vi "NLEISView_Subvi_v15.vi"(0 "Ratio Multiplier":dbl=1.5, 1 "Vk Fitting Algorithm":string(combo)="0", 2 "Char Current (Amps)":dbl=0.067 format="%.5f", 3 "file path (dialog if empty)":path, 4 "LS Program":bool, 5 "Sigma Multiplier":dbl=1.5, 7 "Vk Fitting Tolerance":dbl=0.0001, 9 "Amplitude Run Number":i32, 11 "Frequency Run Number":i32, 12 "Gaussian Window\nParameter (B)":dbl=20.0, 14 "Lookup Table":dbl[][](array[numeric]), 15 "Perturbation Method":bool) -> (6 "Frequency":sgl format="%#.6f", 10 "Fit Coefficients and Noise Ratios":dbl[](array[numeric]) format="%.2f")   [LabVIEW 2018]
uses:
  <vilib>/Analysis/baseanly.llb/Mean (DBL).vi
  <vilib>/Analysis/5stat.llb/RMS (DBL).vi
  <vilib>/Utility/file.llb/Read From Spreadsheet File (DBL).vi
  <vilib>/measure/maspectr.llb/FFT Spectrum (Mag-Phase) for 1 Chan.vi
  <vilib>/Waveform/WDTOps.llb/WDT Get Waveform Time Array DBL.vi
  <vilib>/measure/maspectr.llb/FFT Spectrum (Real-Im) for 1 Chan.vi
  <vilib>/measure/NI_MAPro.lvlib
  <vilib>/Analysis/NI_AALPro.lvlib
  <vilib>/Analysis/NI_AALBase.lvlib
panel:
  out "Voltage (Re and Im), Gaussian FFT vs Fit":dbl[][](graph)
  out "Current (Re and Im), Gaussian FFT vs Fit":dbl[][](graph)
  out "Pre-Filter":dbl[](array[numeric])
  in  "Tab Control":enum32{"Fitting", "Data"}(tab)
  out "sigma noise":dbl format="%.5e"
  out "Current Amplitude":dbl format="%.3f"
  out "V1 Amplitude":dbl format="%.2f"
  out "Current Phase Correction":dbl
  out "Voltage vs Time":cluster{dbl[], dbl[]}(graph)
  out "Current vs Time":cluster{dbl[], dbl[]}(graph)
  out "Current vs Time (Gaussian Window)":waveform(dbl)(graph)
  out "Post-Filter":dbl[](array[numeric])
  out "Voltage Magnitude Hanning FFT":cluster{"f0":dbl, "df":dbl, "magnitude":dbl[]}(graph)
  out "Current Magnitude Hanning FFT":cluster{"f0":dbl, "df":dbl, "magnitude":dbl[]}(graph)
  out "Voltage vs Time (Gaussian Window)":waveform(dbl)(graph)
  # "Fit Voltage Coefficients"
  # "V1 Re\nV1 Im"
  # "V2 Re\nV2 Im"
  # "V3 Re\nV3 Im"
  # "V4 Re\nV4 Im"
  # "V5 Re\nV5 Im"
  # "Flat Baseline Im\nFlat Baseline Re"
  # "Sloped Baseline Origin\nSloped Baseline End"
  # "Appended Array Built As:\n0 - alpha\n1 - V1 Re\n2 - V1 Im\n3 - V2 Re\n4 - V2 Im\n5 - V3 Re\n6 - V3 Im\n7 - V4 Re\n8 - V4 Im\n9 - V5 Re\n10 - V5 Im\n11 - V1 Mag\n12 - V2 Mag\n13 - V3 Mag\n14 - V4 Mag\n15 - V5 Mag\n16 - V1 Phase\n17 - V2 Phase\n18 - V3 Phase\n19 - V4 Phase\n20 - V5 Phase\n21 - alpha Peak/Noise (rms/sigma)\n22 - alpha Noise/Error\n23 - V1 Peak/Noise\n24 - V1 Noise/Error\n25 - V2 Peak/Noise\n26 - V2 Noise/Error\n27 - V3 Peak/Noise\n28 - V3 Noise/Error\n29 - V4 Peak/Noise\n30 - V4 Noise/Error\n31 - V5 Peak/Noise\n32 - V5 Noise/Error"
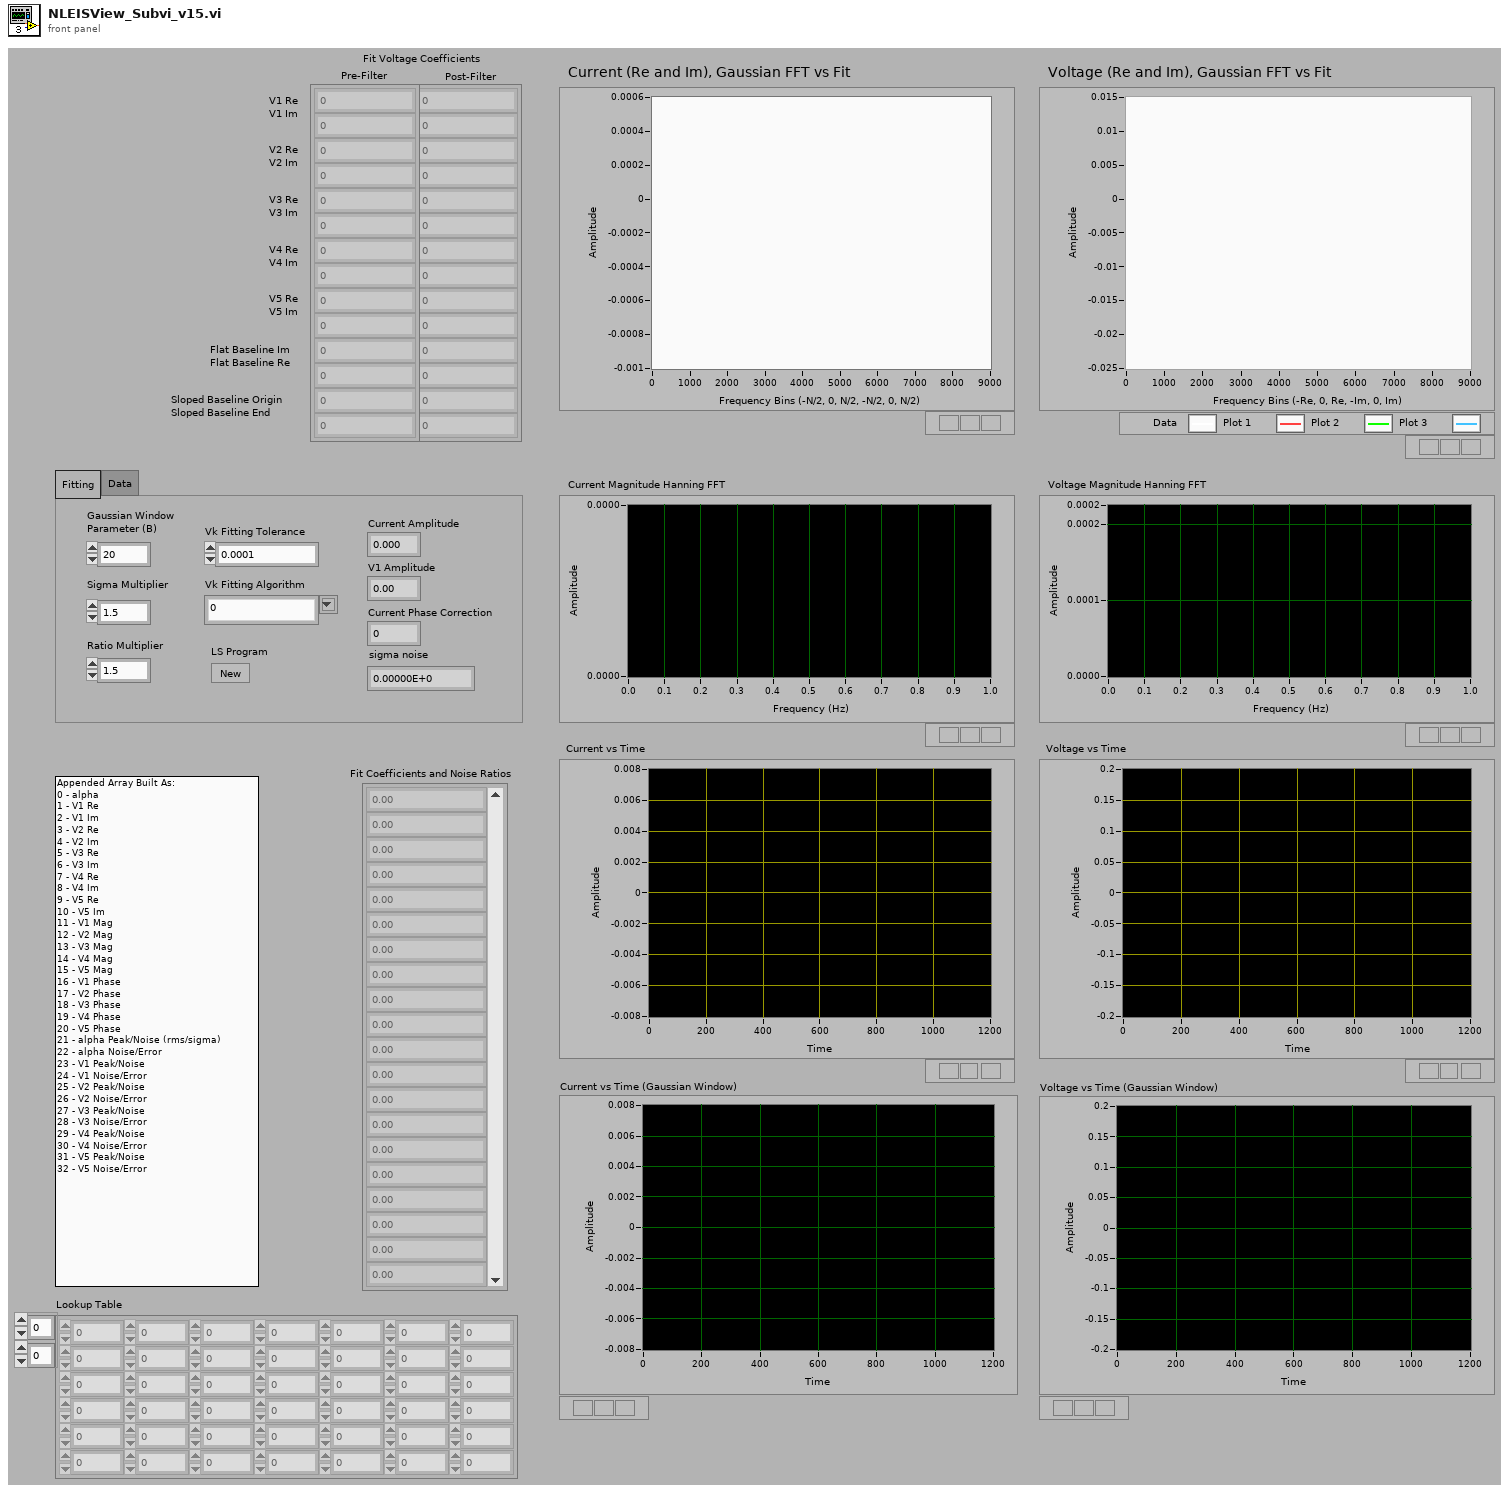
[diagram p1: front panel]
types:
  T1 = enum16{"None ", "Hanning", "Hamming", "Blackman-Harris", "Exact Blackman", "Blackman", "Flat Top", "4 Term B-Harris ", "7 Term B-Harris", "Low Sidelobe"}
  T2 = cluster{"f0":dbl, "df":dbl, "imaginary part":dbl[]}
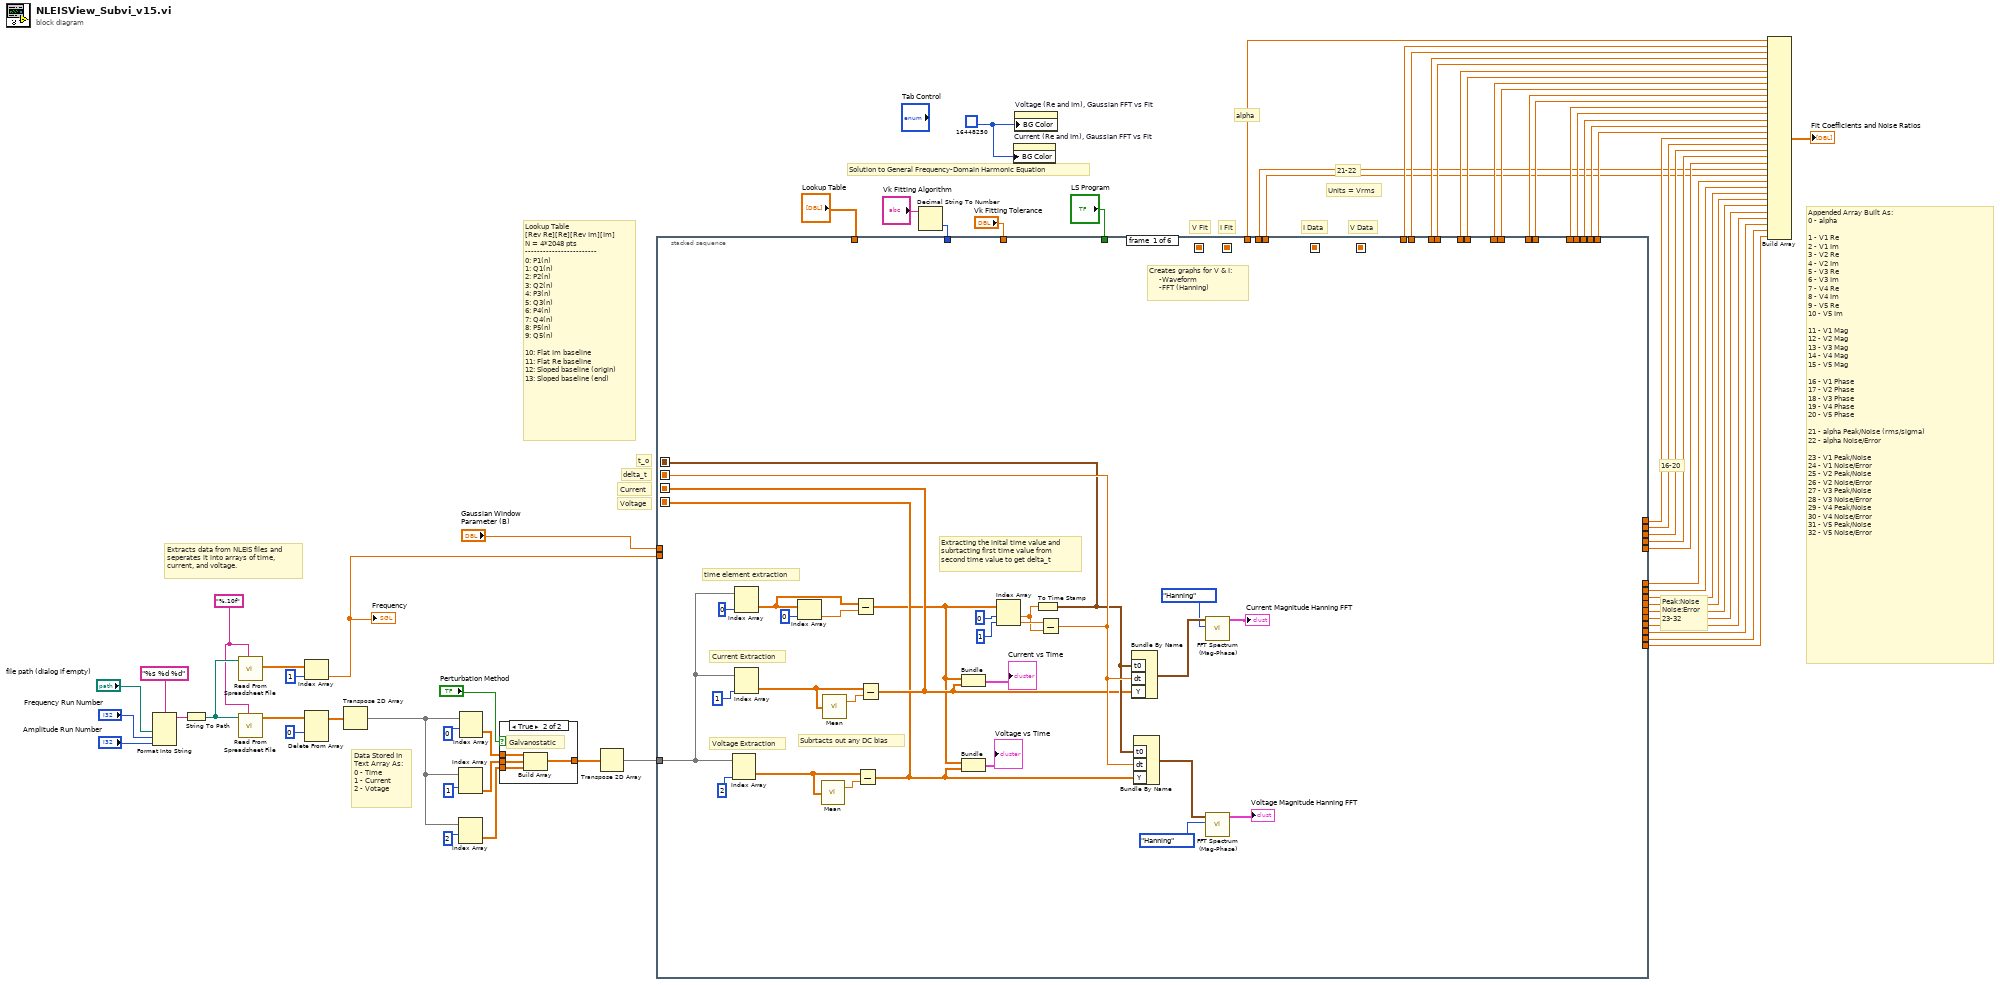
[diagram p0: block diagram]
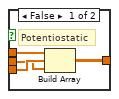
[diagram p2: hidden frame]
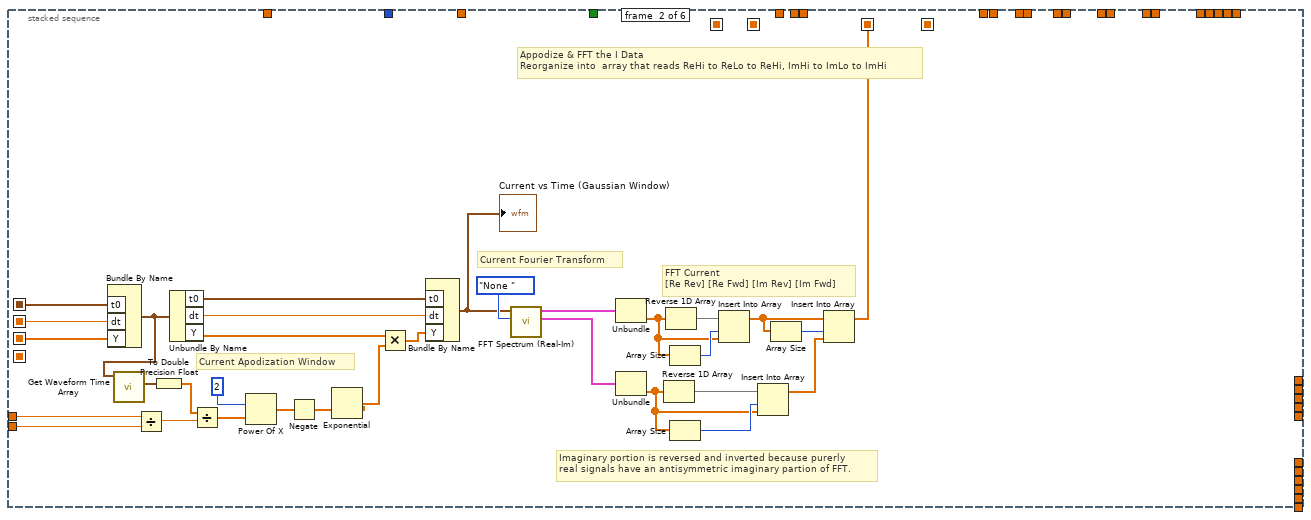
[diagram p3: hidden frame]
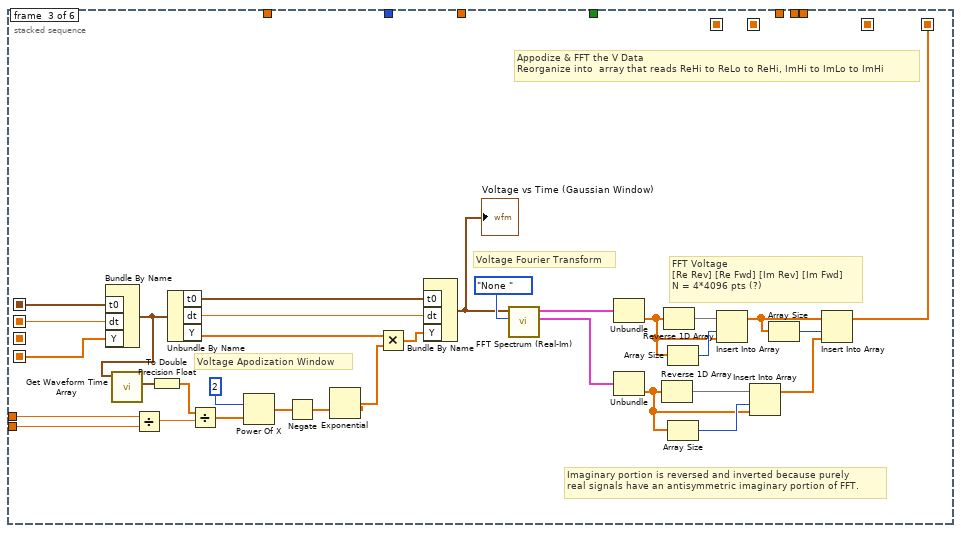
[diagram p4: hidden frame]
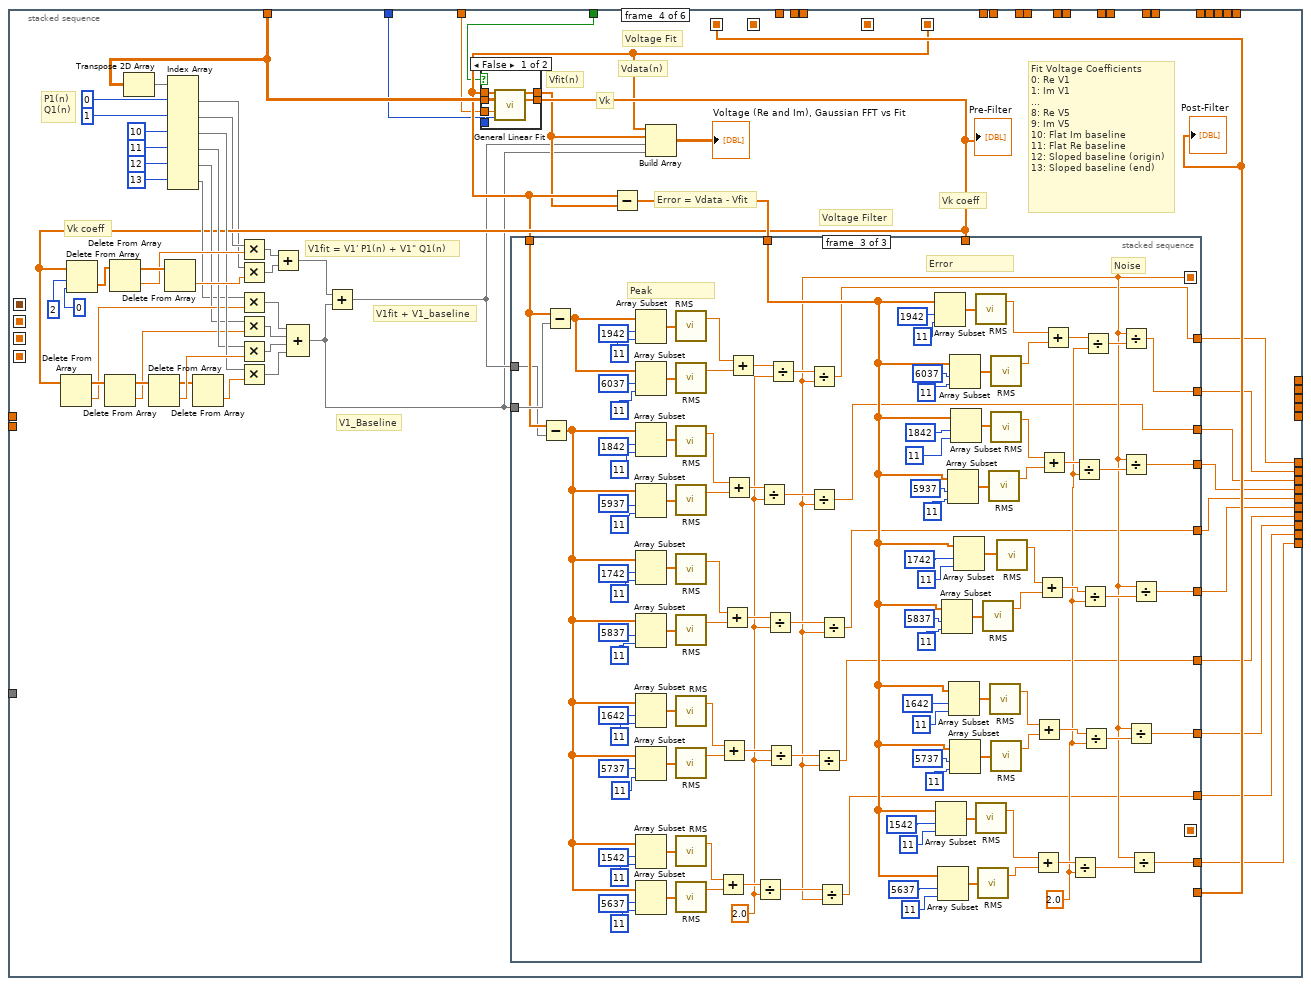
[diagram p5: hidden frame]
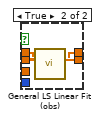
[diagram p6: hidden frame]
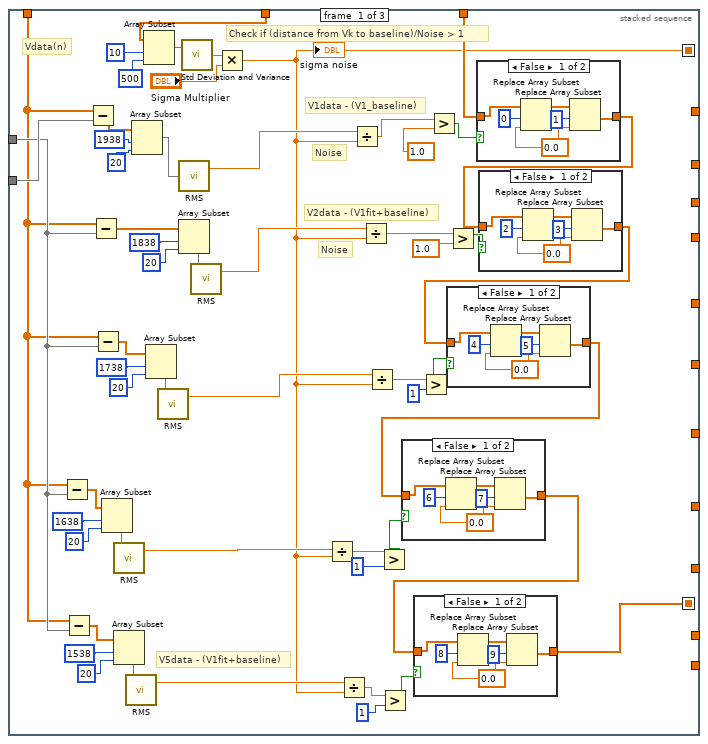
[diagram p7: hidden frame]
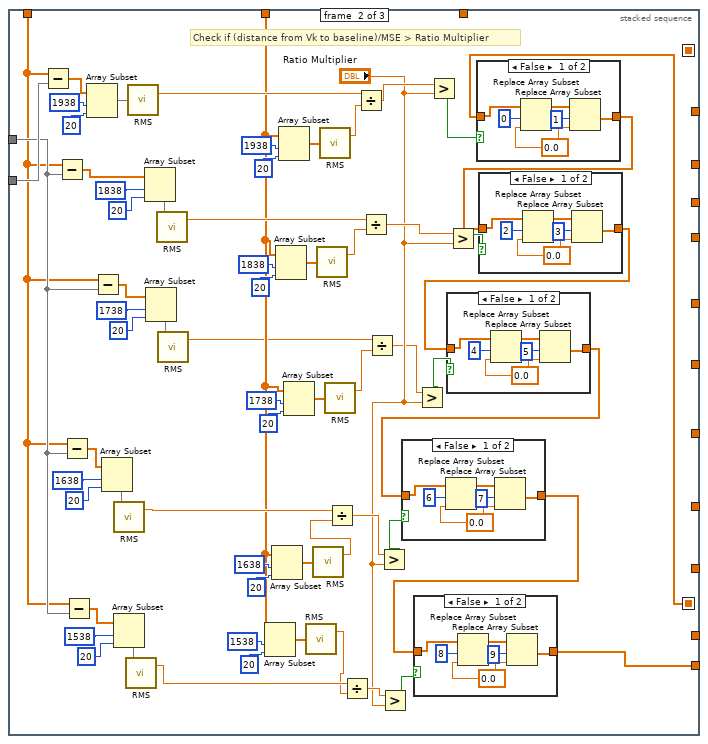
[diagram p13: hidden frame]
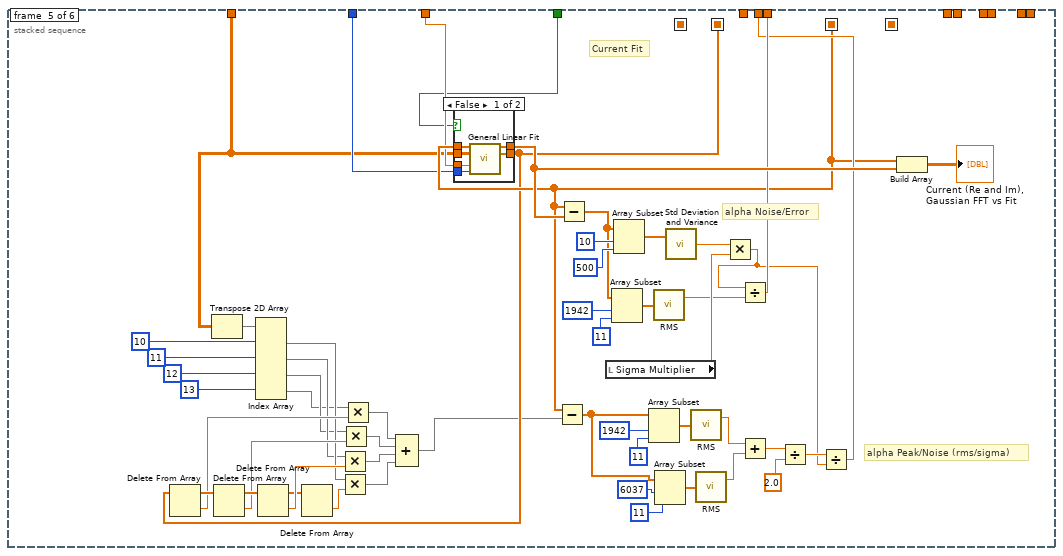
[diagram p19: hidden frame]
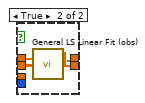
[diagram p20: hidden frame]
diagram:
  w5 = u32 16448250
  w26 = "%.10f" ("format (%.3f)")
  # "alpha"
  # "Lookup Table\n[Rev Re][Re][Rev Im][Im]\nN = 4*2048 pts\n------------------------\n0: P1(n)\n1: Q1(n)\n2: P2(n)\n3: Q2(n)\n4: P3(n)\n5: Q3(n)\n6: P4(n)\n7: Q4(n)\n8: P5(n)\n9: Q5(n)\n\n10: Flat Im baseline\n11: Flat Re baseline\n12: Sloped baseline (origin)\n13: Sloped baseline (end)"
  # "21-22"
  # "16-20"
  # "Peak:Noise\nNoise:Error\n23-32"
  # "Units = Vrms"
  # "Extracts data from NLEIS files and\nseperates it into arrays of time,\ncurrent, and voltage."
  # "Solution to General Frequency-Domain Harmonic Equation"
  # "V Fit"
  # "t_o"
  # "Appended Array Built As:\n0 - alpha\n\n1 - V1 Re\n2 - V1 Im\n3 - V2 Re\n4 - V2 Im\n5 - V3 Re\n6 - V3 Im\n7 - V4 Re\n8 - V4 Im\n9 - V5 Re\n10 - V5 Im\n\n11 - V1 Mag\n12 - V2 Mag\n13 - V3 Mag\n14 - V4 Mag\n15 - V5 Mag\n\n16 - V1 Phase\n17 - V2 Phase\n18 - V3 Phase\n19 - V4 Phase\n20 - V5 Phase\n\n21 - alpha Peak/Noise (rms/sigma)\n22 - alpha Noise/Error\n\n23 - V1 Peak/Noise\n24 - V1 Noise/Error\n25 - V2 Peak/Noise\n26 - V2 Noise/Error\n27 - V3 Peak/Noise\n28 - V3 Noise/Error\n29 - V4 Peak/Noise\n30 - V4 Noise/Error\n31 - V5 Peak/Noise\n32 - V5 Noise/Error"
  # "Data Stored In\nText Array As:\n0 - Time\n1 - Current\n2 - Votage"
  # "I Fit"
  # "V Data"
  # "I Data"
  # "Current"
  # "delta_t"
  # "Voltage"
  n1 = Format Into String(format string="%s %d %d", "file path (dialog if empty)", "Frequency Run Number", "Amplitude Run Number") -> (resulting string=w38:string)  [unwired: 2 in, 1 out]
  n2 = String To Path(string=w38) -> (path=w27:path)
  n3 = call-poly <vilib>:"Read From Spreadsheet File.vi"("format (%.3f)"=w26, "file path (dialog if empty)"=w27) -> ("first row"=w24:dbl[])  [unwired: 5 in, 4 out]
  n4 = call-poly <vilib>:"Read From Spreadsheet File.vi"("format (%.3f)"=w26, "file path (dialog if empty)"=w27) -> ("all rows"=w21:dbl[][])  [unwired: 5 in, 4 out]
  n5 = Index Array(array=w24, index=1) -> (element=w23:dbl)
  "Frequency" <- w23
  n6 = Delete From Array(array=w21, index (row)=0) -> (array with subset deleted=w20:dbl[][])  [unwired: 2 in, 1 out]
  n7 = Transpose 2D Array(2D array=w20) -> (transposed array=w33:dbl[][])
  n8 = Index Array(array=w33, index (row)=1) -> (element=w29:dbl[])  [unwired: 1 in]
  n9 = Index Array(array=w33, index (row)=2) -> (element=w30:dbl[])  [unwired: 1 in]
  n10 = Index Array(array=w33, index (row)=0) -> (element=w32:dbl[])  [unwired: 1 in]
  n11 = case shown="True" "Perturbation Method" {
    tunnel: [w68 w72] -> w61
    tunnel: w32 -> [w67 w71]
    tunnel: w30 -> [w66 w70]
    tunnel: w29 -> [w65 w69]
    frame False {
      # "Potentiostatic"
      n12 = Build Array(w67, w66, w65) -> (w68:dbl[][])
    }
    frame True {
      # "Galvanostatic"
      n13 = Build Array(w71, w69, w70) -> (w72:dbl[][])
    }
  }
  n14 = Transpose 2D Array(2D array=w61) -> (transposed array=w62:dbl[][])
  n15 = Decimal String To Number(string="Vk Fitting Algorithm") -> (number=w2:i32)  [unwired: 2 in, 1 out]
  n16 = stacked-sequence {
    seq-local: [w92 _ _ _ _ _] -> [_ w118 w139 _ _ _]
    seq-local: [w90 _ _ _ _ _] -> [_ w131 _ _ _ _]
    seq-local: [w85 _ _ _ _ _] -> [_ _ w138 _ _ _]
    seq-local: [_ w109 _ _ _ _] -> [_ _ _ _ w568 _]
    seq-local: [_ _ w134 _ _ _] -> [_ _ _ w172 _ _]
    seq-local: [_ _ _ w207 _ _] -> [_ _ _ _ _ w618]
    seq-local: [_ _ _ _ w543 _] -> [_ _ _ _ _ w617]
    seq-local: [w91 _ _ _ _ _] -> [_ w117 w140 _ _ _]
    tunnel: "Gaussian Window\nParameter (B)" -> [_ w120 w137 _ _ _]
    tunnel: [_ _ _ _ _ w652] -> w40
    tunnel: [_ _ _ _ _ w651] -> w41
    tunnel: [_ _ _ _ _ w650] -> w42
    tunnel: [_ _ _ _ _ w649] -> w43
    tunnel: [_ _ _ _ _ w648] -> w44
    tunnel: [_ _ _ _ _ w646] -> w45
    tunnel: [_ _ _ _ _ w645] -> w46
    tunnel: [_ _ _ _ _ w644] -> w47
    tunnel: [_ _ _ _ _ w643] -> w48
    tunnel: [_ _ _ _ _ w642] -> w49
    tunnel: [_ _ _ _ _ w641] -> w50
    tunnel: w62 -> [w97 _ _ _ _ _]
    tunnel: [_ _ _ _ _ w640] -> w51
    tunnel: [_ _ _ _ _ w639] -> w52
    tunnel: [_ _ _ _ _ w638] -> w53
    tunnel: [_ _ _ _ _ w637] -> w54
    tunnel: [_ _ _ _ _ w636] -> w55
    tunnel: [_ _ _ _ _ w635] -> w56
    tunnel: [_ _ _ _ _ w634] -> w57
    tunnel: [_ _ _ _ _ w633] -> w58
    tunnel: [_ _ _ _ _ w632] -> w59
    tunnel: [_ _ _ _ _ w631] -> w60
    tunnel: w23 -> [_ w106 w136 _ _ _]
    tunnel: [_ _ _ _ w574 _] -> w13
    tunnel: [_ _ _ _ w584 _] -> w12
    tunnel: [_ _ _ w205 _ _] -> w19
    tunnel: [_ _ _ w201 _ _] -> w14
    tunnel: [_ _ _ w202 _ _] -> w15
    tunnel: [_ _ _ w204 _ _] -> w16
    tunnel: [_ _ _ w203 _ _] -> w17
    tunnel: [_ _ _ w206 _ _] -> w18
    tunnel: [_ _ _ w200 _ _] -> w11
    tunnel: [_ _ _ w199 _ _] -> w10
    tunnel: [_ _ _ w198 _ _] -> w9
    tunnel: [_ _ _ w197 _ _] -> w8
    tunnel: "Lookup Table" -> [_ _ _ w176 w548 _]
    tunnel: "Vk Fitting Tolerance" -> [_ _ _ w167 w566 _]
    tunnel: w2 -> [_ _ _ w166 w565 _]
    tunnel: "LS Program" -> [_ _ _ w165 w541 _]
    frame #0 {
      # "Extracting the inital time value and\nsubrtacting first time value from\nsecond time value to get delta_t"
      # "Creates graphs for V & I:\n     -Waveform\n     -FFT (Hanning)"
      # "Subrtacts out any DC bias"
      # "Current Extraction"
      # "Voltage Extraction"
      # "time element extraction"
      n17 = Index Array(array=w97, index (col)=2) -> (element=w86:dbl[])  [unwired: 1 in]
      n18 = Index Array(array=w97, index (col)=0) -> (element=w74:dbl[])  [unwired: 1 in]
      n19 = Index Array(array=w97, index (col)=1) -> (element=w89:dbl[])  [unwired: 1 in]
      n20 = Index Array(array=w74, index=0) -> (element=w75:dbl)
      n21 = call-poly <vilib>:"Mean.vi"("X"=w86) -> ("mean"=w87:dbl)  [unwired: 1 out]
      n22 = call-poly <vilib>:"Mean.vi"("X"=w89) -> ("mean"=w88:dbl)  [unwired: 1 out]
      n23 = Subtract(x=w74, y=w75) -> (x-y=w73:dbl[])
      n24 = Subtract(x=w86, y=w87) -> (x-y=w85:dbl[])
      n25 = Subtract(x=w89, y=w88) -> (x-y=w90:dbl[])
      n26 = Bundle(w73, w90) -> (→"Current vs Time":cluster{dbl[], dbl[]})  [unwired: 1 in]
      n27 = Bundle(w73, w85) -> (→"Voltage vs Time":cluster{dbl[], dbl[]})  [unwired: 1 in]
      n28 = Index Array(array=w73, index #1=0 ("index"), index #2=1) -> (element #1=w93:dbl, element #2=w94:dbl)
      n29 = To Time Stamp(1:w93) -> (0:w91:timestamp)
      n30 = Subtract(x=w94, y=w93) -> (x-y=w92:dbl)
      n31 = Bundle By Name("t0"=w91, "dt"=w92, "Y"=w90) -> (w83:waveform(dbl))  [unwired: 1 in]
      n32 = Bundle By Name("t0"=w91, "dt"=w92, "Y"=w85) -> (w79:waveform(dbl))  [unwired: 1 in]
      n33 = call-poly <vilib>:"FFT Spectrum (Mag-Phase).vi"("window"=T1."Hanning", "time signal"=w83) -> ("magnitude"=→"Current Magnitude Hanning FFT":cluster{"f0":dbl, "df":dbl, "magnitude":dbl[]})  [unwired: 5 in, 4 out]
      n34 = call-poly <vilib>:"FFT Spectrum (Mag-Phase).vi"("window"=T1."Hanning", "time signal"=w79) -> ("magnitude"=→"Voltage Magnitude Hanning FFT":cluster{"f0":dbl, "df":dbl, "magnitude":dbl[]})  [unwired: 5 in, 4 out]
    }
    frame #1 {
      # "FFT Current\n[Re Rev] [Re Fwd] [Im Rev] [Im Fwd]"
      # "Appodize & FFT the I Data\nReorganize into  array that reads ReHi to ReLo to ReHi, ImHi to ImLo to ImHi"
      # "Imaginary portion is reversed and inverted because purerly\nreal signals have an antisymmetric imaginary partion of FFT."
      # "Current Apodization Window"
      # "Real 3rd Voltage"
      # "Real 1rst Voltage"
      # "Current Fourier Transform"
      n35 = Bundle By Name("t0"=w117, "dt"=w118, "Y"=w131) -> (w108:waveform(dbl))  [unwired: 1 in]
      n36 = call-poly <vilib>:"Get Waveform Time Array.vi"("waveform in"=w108) -> ("X array"=w107:timestamp[])  [unwired: 9 in, 1 out]
      n37 = Divide(x=w120, y=w106) -> (x/y=w122:dbl)
      n38 = To Double Precision Float(number=w107) -> (double precision float=w121:dbl[])
      n39 = Unbundle By Name(w108) -> ("t0"=w119:timestamp, "dt"=w130:dbl, "Y"=w129:dbl[])
      n40 = Divide(x=w121, y=w122) -> (x/y=w123:dbl[])
      n41 = Power Of X(1:w123, 2:2) -> (0:w128:dbl[])
      n42 = Negate(x=w128) -> (-x=w124:dbl[])
      n43 = Exponential(1:w124) -> (0:w125:dbl[])
      n44 = Multiply(x=w129, y=w125) -> (x*y=w126:dbl[])
      n45 = Bundle By Name("t0"=w119, "dt"=w130, "Y"=w126) -> (w102:waveform(dbl))  [unwired: 1 in]
      "Current vs Time (Gaussian Window)" <- w102
      n46 = call-poly <vilib>:"FFT Spectrum (Real-Im).vi"("window"=T1."None ", "time signal"=w102) -> ("imaginary part"=w110:T2, "real part"=w111:cluster{"f0":dbl, "df":dbl, "real part":dbl[]})  [unwired: 5 in, 3 out]
      n47 = Unbundle(w111) -> ("real part"=w105:dbl[])  [unwired: 2 out]
      n48 = Unbundle(w110) -> ("imaginary part"=w104:dbl[])  [unwired: 2 out]
      n49 = Reverse 1D Array(array=w104) -> (reversed array=w101:dbl[])
      n50 = Reverse 1D Array(array=w105) -> (reversed array=w116:dbl[])
      n51 = Array Size(array=w105) -> (size(s)=w114:i32)
      n52 = Array Size(array=w104) -> (size(s)=w115:i32)
      n53 = Insert Into Array(array=w116, index=w114, new element=w105) -> (w103:dbl[])
      n54 = Insert Into Array(array=w101, index=w115, new element=w104) -> (w112:dbl[])
      n55 = Array Size(array=w103) -> (size(s)=w113:i32)
      n56 = Insert Into Array(array=w103, index=w113, new element=w112) -> (w109:dbl[])
    }
    frame #2 {
      # "FFT Voltage\n[Re Rev] [Re Fwd] [Im Rev] [Im Fwd]\nN = 4*4096 pts (?)"
      # "Appodize & FFT the V Data\nReorganize into  array that reads ReHi to ReLo to ReHi, ImHi to ImLo to ImHi"
      # "Imaginary portion is reversed and inverted because purely\nreal signals have an antisymmetric imaginary portion of FFT."
      # "Voltage Apodization Window"
      # "Voltage Fourier Transform"
      n57 = Bundle By Name("t0"=w140, "dt"=w139, "Y"=w138) -> (w145:waveform(dbl))  [unwired: 1 in]
      n58 = call-poly <vilib>:"Get Waveform Time Array.vi"("waveform in"=w145) -> ("X array"=w144:timestamp[])  [unwired: 9 in, 1 out]
      n59 = Divide(x=w137, y=w136) -> (x/y=w155:dbl)
      n60 = To Double Precision Float(number=w144) -> (double precision float=w154:dbl[])
      n61 = Unbundle By Name(w145) -> ("t0"=w153:timestamp, "dt"=w163:dbl, "Y"=w162:dbl[])
      n62 = Divide(x=w154, y=w155) -> (x/y=w156:dbl[])
      n63 = Power Of X(1:w156, 2:2) -> (0:w161:dbl[])
      n64 = Negate(x=w161) -> (-x=w157:dbl[])
      n65 = Exponential(1:w157) -> (0:w158:dbl[])
      n66 = Multiply(x=w162, y=w158) -> (x*y=w159:dbl[])
      n67 = Bundle By Name("t0"=w153, "dt"=w163, "Y"=w159) -> (w135:waveform(dbl))  [unwired: 1 in]
      "Voltage vs Time (Gaussian Window)" <- w135
      n68 = call-poly <vilib>:"FFT Spectrum (Real-Im).vi"("window"=T1."None ", "time signal"=w135) -> ("imaginary part"=w146:T2, "real part"=w147:cluster{"f0":dbl, "df":dbl, "real part":dbl[]})  [unwired: 5 in, 3 out]
      n69 = Unbundle(w147) -> ("real part"=w143:dbl[])  [unwired: 2 out]
      n70 = Unbundle(w146) -> ("imaginary part"=w142:dbl[])  [unwired: 2 out]
      n71 = Reverse 1D Array(array=w142) -> (reversed array=w133:dbl[])
      n72 = Reverse 1D Array(array=w143) -> (reversed array=w152:dbl[])
      n73 = Array Size(array=w143) -> (size(s)=w150:i32)
      n74 = Array Size(array=w142) -> (size(s)=w151:i32)
      n75 = Insert Into Array(array=w152, index=w150, new element=w143) -> (w141:dbl[])
      n76 = Insert Into Array(array=w133, index=w151, new element=w142) -> (w148:dbl[])
      n77 = Array Size(array=w141) -> (size(s)=w149:i32)
      n78 = Insert Into Array(array=w141, index=w149, new element=w148) -> (w134:dbl[])
    }
    frame #3 {
      # "Vk"
      # "Vfit(n)"
      # "Vdata(n)"
      # "V1_Baseline"
      # "P1(n)\nQ1(n)"
      # "Vk coeff"
      # "Fit Voltage Coefficients\n0: Re V1\n1: Im V1\n...\n8: Re V5\n9: Im V5\n10: Flat Im baseline\n11: Flat Re baseline\n12: Sloped baseline (origin)\n13: Sloped baseline (end)"
      # "V1fit = V1' P1(n) + V1\" Q1(n)"
      # "Vk coeff"
      # "Error = Vdata - Vfit"
      # "Voltage Filter"
      # "Voltage Fit"
      # "V1fit + V1_baseline"
      n79 = Transpose 2D Array(2D array=w176) -> (transposed array=w175:dbl[][])
      n80 = Index Array(array=w175, index (row) #1=0, index (row) #2=1, index (row) #3=10, index (row) #4=11, index (row) #5=12, index (row) #6=13) -> (element #1=w173:dbl[], element #2=w174:dbl[], element #3=w188:dbl[], element #4=w187:dbl[], element #5=w184:dbl[], element #6=w183:dbl[])  [unwired: 6 in]
      n81 = case shown="False" w165 {
        tunnel: [w225 w227] -> w177
        tunnel: w176 -> [w224 w229]
        tunnel: w172 -> [w223 w228]
        tunnel: [w222 w226] -> w171
        tunnel: w167 -> [w221 _]
        tunnel: w166 -> [w220 _]
        frame False {
          n82 = call <vilib>:"General Linear Fit.vi"("Y"=w223, "H"=w224, "tolerance"=w221, "method"=w220) -> ("Best Fit"=w222:dbl[], "Coefficients"=w225:dbl[])  [unwired: 6 in, 4 out]
        }
        frame True {
          n83 = call <vilib>:"General LS Linear Fit (obs).vi"("H"=w229, "Y"=w228) -> ("Coefficients"=w227:dbl[], "Best Fit"=w226:dbl[])  [unwired: 3 in, 3 out]
        }
      }
      "Pre-Filter" <- w177
      n84 = Delete From Array(array=w177) -> (deleted portion=w185:dbl, array with subset deleted=w190:dbl[])  [unwired: 2 in]
      n85 = Delete From Array(array=w177, length=2 ("index"), index=0 ("length")) -> (deleted portion=w208:dbl[])  [unwired: 1 out]
      n86 = Delete From Array(array=w190) -> (deleted portion=w186:dbl, array with subset deleted=w189:dbl[])  [unwired: 2 in]
      n87 = Delete From Array(array=w208) -> (deleted portion=w214:dbl, array with subset deleted=w219:dbl[])  [unwired: 2 in]
      n88 = Delete From Array(array=w189) -> (deleted portion=w212:dbl, array with subset deleted=w211:dbl[])  [unwired: 2 in]
      n89 = Delete From Array(array=w219) -> (deleted portion=w215:dbl)  [unwired: 2 in, 1 out]
      n90 = Delete From Array(array=w211) -> (deleted portion=w210:dbl)  [unwired: 2 in, 1 out]
      n91 = Multiply(x=w174, y=w214) -> (x*y=w217:dbl[])
      n92 = Multiply(x=w173, y=w215) -> (x*y=w218:dbl[])
      n93 = Multiply(x=w183, y=w185) -> (x*y=w182:dbl[])
      n94 = Multiply(x=w184, y=w186) -> (x*y=w181:dbl[])
      n95 = Multiply(x=w187, y=w212) -> (x*y=w180:dbl[])
      n96 = Multiply(x=w188, y=w210) -> (x*y=w179:dbl[])
      n97 = Add(x=w217, y=w218) -> (x+y=w213:dbl[])
      n98 = Compound Arithmetic op=ADD(w182, w181, w180, w179) -> (w169:dbl[])
      n99 = Add(x=w213, y=w169) -> (x+y=w170:dbl[])
      n100 = Subtract(x=w172, y=w171) -> (x-y=w178:dbl[])
      n101 = stacked-sequence {
        seq-local: [w248 _ _] -> [_ w346 _]
        seq-local: [w230 _ _] -> [_ _ w432]
        tunnel: w177 -> [w284 _ _]
        tunnel: w178 -> [w247 w329 w439]
        tunnel: [_ w345 _] -> w207
        tunnel: w172 -> [w238 w348 w509]
        tunnel: w169 -> [w246 w356 w513]
        tunnel: w170 -> [w244 w354 w508]
        tunnel: [_ _ w430] -> w206
        tunnel: [_ _ w431] -> w205
        tunnel: [_ _ w429] -> w203
        tunnel: [_ _ w428] -> w204
        tunnel: [_ _ w427] -> w202
        tunnel: [_ _ w426] -> w201
        tunnel: [_ _ w425] -> w200
        tunnel: [_ _ w424] -> w199
        tunnel: [_ _ w423] -> w198
        tunnel: [_ _ w422] -> w197
        frame #0 {
          # "V5data - (V1fit+baseline)"
          # "Noise"
          # "V2data - (V1fit+baseline)"
          # "Noise"
          # "Vdata(n)"
          # "V1data - (V1_baseline)"
          # "Check if (distance from Vk to baseline)/Noise > 1"
          n102 = Subtract(x=w238, y=w244) -> (x-y=w241:dbl[])
          n103 = Subtract(x=w238, y=w244) -> (x-y=w240:dbl[])
          n104 = Subtract(x=w238, y=w246) -> (x-y=w245:dbl[])
          n105 = Subtract(x=w238, y=w244) -> (x-y=w243:dbl[])
          n106 = Subtract(x=w238, y=w244) -> (x-y=w242:dbl[])
          n107 = Array Subset(array=w241, index=1638, length=20) -> (w269:dbl[])
          n108 = call-poly <vilib>:"RMS.vi"("X"=w269) -> ("rms value"=w235:dbl)  [unwired: 1 out]
          n109 = Array Subset(array=w240, index=1538, length=20) -> (w264:dbl[])
          n110 = call-poly <vilib>:"RMS.vi"("X"=w264) -> ("rms value"=w231:dbl)  [unwired: 1 out]
          n111 = Array Subset(array=w245, index=1938, length=20) -> (w261:dbl[])
          n112 = Array Subset(array=w247, index=10, length=500) -> (w236:dbl[])
          n113 = Array Subset(array=w242, index=1738, length=20) -> (w273:dbl[])
          n114 = call-poly <vilib>:"RMS.vi"("X"=w273) -> ("rms value"=w232:dbl)  [unwired: 1 out]
          n115 = call-poly <vilib>:"RMS.vi"("X"=w261) -> ("rms value"=w259:dbl)  [unwired: 1 out]
          n116 = Array Subset(array=w243, index=1838, length=20) -> (w277:dbl[])
          n117 = call <vilib>:"Std Deviation and Variance.vi"("X"=w236) -> ("standard deviation"=w237:dbl)  [unwired: 1 in, 2 out]
          n118 = call-poly <vilib>:"RMS.vi"("X"=w277) -> ("rms value"=w233:dbl)  [unwired: 1 out]
          n119 = Multiply(x=w237, y="Sigma Multiplier") -> (x*y=w230:dbl)
          "sigma noise" <- w230
          n120 = Divide(x=w235, y=w230) -> (x/y=w253:dbl)
          n121 = Divide(x=w231, y=w230) -> (x/y=w250:dbl)
          n122 = Divide(x=w259, y=w230) -> (x/y=w258:dbl)
          n123 = Divide(x=w233, y=w230) -> (x/y=w255:dbl)
          n124 = Divide(x=w232, y=w230) -> (x/y=w252:dbl)
          n125 = Greater?(x=w253, y=1) -> (0:w268:bool)
          n126 = Greater?(x=w250, y=1) -> (0:w263:bool)
          n127 = Greater?(x=w252, y=1) -> (0:w239:bool)
          n128 = Greater?(x=w258, y=1.0) -> (0:w285:bool)
          n129 = Greater?(x=w255, y=1.0) -> (0:w276:bool)
          n130 = case shown="False" w285 {
            tunnel: w284 -> [w319 w320]
            tunnel: [w314 w320] -> w283
            frame False {
              w316 = 0.0 ("new element/subarray")
              n131 = Replace Array Subset(array=w319, new element=w316, index=0) -> (w317:dbl[])
              n132 = Replace Array Subset(array=w317, new element=w316, index=1) -> (w314:dbl[])
            }
            frame True {
            }
          }
          n133 = case shown="False" w276 {
            tunnel: w283 -> [w312 w313]
            tunnel: [w307 w313] -> w272
            frame False {
              w309 = 0.0 ("new element/subarray")
              n134 = Replace Array Subset(array=w312, new element=w309, index=2) -> (w310:dbl[])
              n135 = Replace Array Subset(array=w310, new element=w309, index=3) -> (w307:dbl[])
            }
            frame True {
            }
          }
          n136 = case shown="False" w239 {
            tunnel: w272 -> [w305 w306]
            tunnel: [w300 w306] -> w267
            frame False {
              w302 = 0.0 ("new element/subarray")
              n137 = Replace Array Subset(array=w305, new element=w302, index=4) -> (w303:dbl[])
              n138 = Replace Array Subset(array=w303, new element=w302, index=5) -> (w300:dbl[])
            }
            frame True {
            }
          }
          n139 = case shown="False" w268 {
            tunnel: w267 -> [w298 w299]
            tunnel: [w293 w299] -> w262
            frame False {
              w295 = 0.0 ("new element/subarray")
              n140 = Replace Array Subset(array=w298, new element=w295, index=6) -> (w296:dbl[])
              n141 = Replace Array Subset(array=w296, new element=w295, index=7) -> (w293:dbl[])
            }
            frame True {
            }
          }
          n142 = case shown="False" w263 {
            tunnel: w262 -> [w291 w292]
            tunnel: [w286 w292] -> w248
            frame False {
              w288 = 0.0 ("new element/subarray")
              n143 = Replace Array Subset(array=w291, new element=w288, index=8) -> (w289:dbl[])
              n144 = Replace Array Subset(array=w289, new element=w288, index=9) -> (w286:dbl[])
            }
            frame True {
            }
          }
        }
        frame #1 {
          # "Check if (distance from Vk to baseline)/MSE > Ratio Multiplier"
          n145 = Subtract(x=w348, y=w356) -> (x-y=w355:dbl[])
          n146 = Subtract(x=w348, y=w354) -> (x-y=w353:dbl[])
          n147 = Subtract(x=w348, y=w354) -> (x-y=w351:dbl[])
          n148 = Subtract(x=w348, y=w354) -> (x-y=w350:dbl[])
          n149 = Array Subset(array=w355, index=1938, length=20) -> (w365:dbl[])
          n150 = Subtract(x=w348, y=w354) -> (x-y=w352:dbl[])
          n151 = Array Subset(array=w351, index=1638, length=20) -> (w373:dbl[])
          n152 = call-poly <vilib>:"RMS.vi"("X"=w373) -> ("rms value"=w347:dbl)  [unwired: 1 out]
          n153 = Array Subset(array=w350, index=1538, length=20) -> (w368:dbl[])
          n154 = call-poly <vilib>:"RMS.vi"("X"=w368) -> ("rms value"=w358:dbl)  [unwired: 1 out]
          n155 = call-poly <vilib>:"RMS.vi"("X"=w365) -> ("rms value"=w363:dbl)  [unwired: 1 out]
          n156 = Array Subset(array=w353, index=1838, length=20) -> (w381:dbl[])
          n157 = Array Subset(array=w352, index=1738, length=20) -> (w377:dbl[])
          n158 = call-poly <vilib>:"RMS.vi"("X"=w381) -> ("rms value"=w361:dbl)  [unwired: 1 out]
          n159 = call-poly <vilib>:"RMS.vi"("X"=w377) -> ("rms value"=w326:dbl)  [unwired: 1 out]
          n160 = Array Subset(array=w329, index=1538, length=20) -> (w330:dbl[])
          n161 = Array Subset(array=w329, index=1638, length=20) -> (w333:dbl[])
          n162 = Array Subset(array=w329, index=1838, length=20) -> (w339:dbl[])
          n163 = Array Subset(array=w329, index=1938, length=20) -> (w342:dbl[])
          n164 = Array Subset(array=w329, index=1738, length=20) -> (w336:dbl[])
          n165 = call-poly <vilib>:"RMS.vi"("X"=w330) -> ("rms value"=w325:dbl)  [unwired: 1 out]
          n166 = call-poly <vilib>:"RMS.vi"("X"=w333) -> ("rms value"=w324:dbl)  [unwired: 1 out]
          n167 = call-poly <vilib>:"RMS.vi"("X"=w339) -> ("rms value"=w322:dbl)  [unwired: 1 out]
          n168 = call-poly <vilib>:"RMS.vi"("X"=w342) -> ("rms value"=w321:dbl)  [unwired: 1 out]
          n169 = call-poly <vilib>:"RMS.vi"("X"=w336) -> ("rms value"=w323:dbl)  [unwired: 1 out]
          n170 = Divide(x=w347, y=w324) -> (x/y=w359:dbl)
          n171 = Divide(x=w358, y=w325) -> (x/y=w357:dbl)
          n172 = Divide(x=w363, y=w321) -> (x/y=w362:dbl)
          n173 = Divide(x=w361, y=w322) -> (x/y=w360:dbl)
          n174 = Divide(x=w326, y=w323) -> (x/y=w327:dbl)
          n175 = Greater?(x=w359, y="Ratio Multiplier") -> (0:w372:bool)
          n176 = Greater?(x=w357, y="Ratio Multiplier") -> (0:w367:bool)
          n177 = Greater?(x=w327, y="Ratio Multiplier") -> (0:w349:bool)
          n178 = Greater?(x=w362, y="Ratio Multiplier") -> (0:w386:bool)
          n179 = Greater?(x=w360, y="Ratio Multiplier") -> (0:w380:bool)
          n180 = case shown="False" w386 {
            tunnel: w346 -> [w420 w421]
            tunnel: [w415 w421] -> w385
            frame False {
              w417 = 0.0 ("new element/subarray")
              n181 = Replace Array Subset(array=w420, new element=w417, index=0) -> (w418:dbl[])
              n182 = Replace Array Subset(array=w418, new element=w417, index=1) -> (w415:dbl[])
            }
            frame True {
            }
          }
          n183 = case shown="False" w380 {
            tunnel: w385 -> [w413 w414]
            tunnel: [w408 w414] -> w376
            frame False {
              w410 = 0.0 ("new element/subarray")
              n184 = Replace Array Subset(array=w413, new element=w410, index=2) -> (w411:dbl[])
              n185 = Replace Array Subset(array=w411, new element=w410, index=3) -> (w408:dbl[])
            }
            frame True {
            }
          }
          n186 = case shown="False" w349 {
            tunnel: w376 -> [w406 w407]
            tunnel: [w401 w407] -> w371
            frame False {
              w403 = 0.0 ("new element/subarray")
              n187 = Replace Array Subset(array=w406, new element=w403, index=4) -> (w404:dbl[])
              n188 = Replace Array Subset(array=w404, new element=w403, index=5) -> (w401:dbl[])
            }
            frame True {
            }
          }
          n189 = case shown="False" w372 {
            tunnel: w371 -> [w399 w400]
            tunnel: [w394 w400] -> w366
            frame False {
              w396 = 0.0 ("new element/subarray")
              n190 = Replace Array Subset(array=w399, new element=w396, index=6) -> (w397:dbl[])
              n191 = Replace Array Subset(array=w397, new element=w396, index=7) -> (w394:dbl[])
            }
            frame True {
            }
          }
          n192 = case shown="False" w367 {
            tunnel: w366 -> [w392 w393]
            tunnel: [w387 w393] -> w345
            frame False {
              w389 = 0.0 ("new element/subarray")
              n193 = Replace Array Subset(array=w392, new element=w389, index=8) -> (w390:dbl[])
              n194 = Replace Array Subset(array=w390, new element=w389, index=9) -> (w387:dbl[])
            }
            frame True {
            }
          }
        }
        frame #2 {
          w433 = 2.0
          w489 = 2.0
          # "Error"
          # "Noise"
          # "Peak"
          n195 = Subtract(x=w509, y=w508) -> (x-y=w506:dbl[])
          n196 = Subtract(x=w509, y=w513) -> (x-y=w507:dbl[])
          n197 = Array Subset(array=w507, index=1942, length=11) -> (w527:dbl[])
          n198 = Array Subset(array=w507, index=6037, length=11) -> (w524:dbl[])
          n199 = Array Subset(array=w506, index=1842, length=11) -> (w537:dbl[])
          n200 = Array Subset(array=w506, index=5937, length=11) -> (w521:dbl[])
          n201 = Array Subset(array=w506, index=1742, length=11) -> (w534:dbl[])
          n202 = Array Subset(array=w506, index=5837, length=11) -> (w518:dbl[])
          n203 = Array Subset(array=w506, index=1642, length=11) -> (w531:dbl[])
          n204 = Array Subset(array=w506, index=5737, length=11) -> (w515:dbl[])
          n205 = Array Subset(array=w506, index=1542, length=11) -> (w528:dbl[])
          n206 = Array Subset(array=w506, index=5637, length=11) -> (w510:dbl[])
          n207 = call-poly <vilib>:"RMS.vi"("X"=w527) -> ("rms value"=w505:dbl)  [unwired: 1 out]
          n208 = call-poly <vilib>:"RMS.vi"("X"=w524) -> ("rms value"=w504:dbl)  [unwired: 1 out]
          n209 = call-poly <vilib>:"RMS.vi"("X"=w537) -> ("rms value"=w503:dbl)  [unwired: 1 out]
          n210 = call-poly <vilib>:"RMS.vi"("X"=w521) -> ("rms value"=w502:dbl)  [unwired: 1 out]
          n211 = call-poly <vilib>:"RMS.vi"("X"=w534) -> ("rms value"=w498:dbl)  [unwired: 1 out]
          n212 = call-poly <vilib>:"RMS.vi"("X"=w518) -> ("rms value"=w497:dbl)  [unwired: 1 out]
          n213 = call-poly <vilib>:"RMS.vi"("X"=w531) -> ("rms value"=w495:dbl)  [unwired: 1 out]
          n214 = call-poly <vilib>:"RMS.vi"("X"=w515) -> ("rms value"=w494:dbl)  [unwired: 1 out]
          n215 = call-poly <vilib>:"RMS.vi"("X"=w528) -> ("rms value"=w492:dbl)  [unwired: 1 out]
          n216 = call-poly <vilib>:"RMS.vi"("X"=w510) -> ("rms value"=w491:dbl)  [unwired: 1 out]
          n217 = Add(x=w492, y=w491) -> (x+y=w490:dbl)
          n218 = Add(x=w495, y=w494) -> (x+y=w493:dbl)
          n219 = Add(x=w498, y=w497) -> (x+y=w496:dbl)
          n220 = Add(x=w503, y=w502) -> (x+y=w501:dbl)
          n221 = Add(x=w505, y=w504) -> (x+y=w500:dbl)
          n222 = Divide(x=w490, y=w489) -> (x/y=w488:dbl)
          n223 = Divide(x=w501, y=w489) -> (x/y=w487:dbl)
          n224 = Divide(x=w496, y=w489) -> (x/y=w486:dbl)
          n225 = Divide(x=w493, y=w489) -> (x/y=w485:dbl)
          n226 = Divide(x=w500, y=w489) -> (x/y=w499:dbl)
          n227 = Divide(x=w499, y=w432) -> (x/y=w431:dbl)
          n228 = Divide(x=w487, y=w432) -> (x/y=w429:dbl)
          n229 = Divide(x=w485, y=w432) -> (x/y=w425:dbl)
          n230 = Divide(x=w488, y=w432) -> (x/y=w423:dbl)
          n231 = Divide(x=w486, y=w432) -> (x/y=w427:dbl)
          n232 = Array Subset(array=w439, index=1942, length=11) -> (w471:dbl[])
          n233 = Array Subset(array=w439, index=1542, length=11) -> (w472:dbl[])
          n234 = Array Subset(array=w439, index=5637, length=11) -> (w455:dbl[])
          n235 = Array Subset(array=w439, index=5837, length=11) -> (w462:dbl[])
          n236 = Array Subset(array=w439, index=5937, length=11) -> (w465:dbl[])
          n237 = Array Subset(array=w439, index=1642, length=11) -> (w475:dbl[])
          n238 = Array Subset(array=w439, index=6037, length=11) -> (w468:dbl[])
          n239 = Array Subset(array=w439, index=5737, length=11) -> (w459:dbl[])
          n240 = Array Subset(array=w439, index=1842, length=11) -> (w481:dbl[])
          n241 = Array Subset(array=w439, index=1742, length=11) -> (w478:dbl[])
          n242 = call-poly <vilib>:"RMS.vi"("X"=w471) -> ("rms value"=w454:dbl)  [unwired: 1 out]
          n243 = call-poly <vilib>:"RMS.vi"("X"=w472) -> ("rms value"=w442:dbl)  [unwired: 1 out]
          n244 = call-poly <vilib>:"RMS.vi"("X"=w455) -> ("rms value"=w441:dbl)  [unwired: 1 out]
          n245 = call-poly <vilib>:"RMS.vi"("X"=w462) -> ("rms value"=w447:dbl)  [unwired: 1 out]
          n246 = call-poly <vilib>:"RMS.vi"("X"=w465) -> ("rms value"=w451:dbl)  [unwired: 1 out]
          n247 = call-poly <vilib>:"RMS.vi"("X"=w475) -> ("rms value"=w445:dbl)  [unwired: 1 out]
          n248 = call-poly <vilib>:"RMS.vi"("X"=w468) -> ("rms value"=w453:dbl)  [unwired: 1 out]
          n249 = call-poly <vilib>:"RMS.vi"("X"=w481) -> ("rms value"=w452:dbl)  [unwired: 1 out]
          n250 = call-poly <vilib>:"RMS.vi"("X"=w459) -> ("rms value"=w444:dbl)  [unwired: 1 out]
          n251 = call-poly <vilib>:"RMS.vi"("X"=w478) -> ("rms value"=w448:dbl)  [unwired: 1 out]
          n252 = Add(x=w442, y=w441) -> (x+y=w440:dbl)
          n253 = Add(x=w445, y=w444) -> (x+y=w443:dbl)
          n254 = Add(x=w448, y=w447) -> (x+y=w446:dbl)
          n255 = Add(x=w452, y=w451) -> (x+y=w450:dbl)
          n256 = Add(x=w454, y=w453) -> (x+y=w449:dbl)
          n257 = Divide(x=w440, y=w433) -> (x/y=w434:dbl)
          n258 = Divide(x=w450, y=w433) -> (x/y=w437:dbl)
          n259 = Divide(x=w446, y=w433) -> (x/y=w436:dbl)
          n260 = Divide(x=w443, y=w433) -> (x/y=w435:dbl)
          n261 = Divide(x=w449, y=w433) -> (x/y=w438:dbl)
          n262 = Divide(x=w432, y=w438) -> (x/y=w430:dbl)
          n263 = Divide(x=w432, y=w437) -> (x/y=w428:dbl)
          n264 = Divide(x=w432, y=w435) -> (x/y=w424:dbl)
          n265 = Divide(x=w432, y=w434) -> (x/y=w422:dbl)
          n266 = Divide(x=w432, y=w436) -> (x/y=w426:dbl)
        }
      }
      "Post-Filter" <- w207
      n267 = Build Array(w172, w171, w170, w169) -> (→"Voltage (Re and Im), Gaussian FFT vs Fit":dbl[][])
    }
    frame #4 {
      # "alpha Noise/Error"
      # "alpha Peak/Noise (rms/sigma)"
      # "Current Fit"
      n268 = Transpose 2D Array(2D array=w548) -> (transposed array=w549:dbl[][])
      n269 = Index Array(array=w549, index (row) #1=10, index (row) #2=11, index (row) #3=12, index (row) #4=13) -> (element #1=w547:dbl[], element #2=w546:dbl[], element #3=w545:dbl[], element #4=w544:dbl[])  [unwired: 4 in]
      n270 = case shown="False" w541 {
        tunnel: [w600 w601] -> w592
        tunnel: w568 -> [w599 w603]
        tunnel: w566 -> [w598 _]
        tunnel: w565 -> [w597 _]
        tunnel: w548 -> [w596 w604]
        tunnel: [w595 w602] -> w543
        frame False {
          n271 = call <vilib>:"General Linear Fit.vi"("Y"=w599, "H"=w596, "tolerance"=w598, "method"=w597) -> ("Best Fit"=w600:dbl[], "Coefficients"=w595:dbl[])  [unwired: 6 in, 4 out]
        }
        frame True {
          n272 = call <vilib>:"General LS Linear Fit (obs).vi"("H"=w604, "Y"=w603) -> ("Coefficients"=w602:dbl[], "Best Fit"=w601:dbl[])  [unwired: 3 in, 3 out]
        }
      }
      n273 = Delete From Array(array=w543) -> (deleted portion=w554:dbl, array with subset deleted=w557:dbl[])  [unwired: 2 in]
      n274 = Delete From Array(array=w557) -> (deleted portion=w555:dbl, array with subset deleted=w556:dbl[])  [unwired: 2 in]
      n275 = Delete From Array(array=w556) -> (deleted portion=w564:dbl, array with subset deleted=w563:dbl[])  [unwired: 2 in]
      n276 = Delete From Array(array=w563) -> (deleted portion=w562:dbl)  [unwired: 2 in, 1 out]
      n277 = Multiply(x=w546, y=w564) -> (x*y=w551:dbl[])
      n278 = Multiply(x=w547, y=w562) -> (x*y=w550:dbl[])
      n279 = Multiply(x=w545, y=w555) -> (x*y=w552:dbl[])
      n280 = Multiply(x=w544, y=w554) -> (x*y=w553:dbl[])
      n281 = Compound Arithmetic op=ADD(w553, w552, w551, w550) -> (w542:dbl[])
      n282 = Subtract(x=w568, y=w542) -> (x-y=w578:dbl[])
      n283 = Subtract(x=w568, y=w592) -> (x-y=w589:dbl[])
      n284 = local read "Sigma Multiplier"() -> (w585:dbl)
      n285 = Array Subset(array=w589, index=1942, length=11) -> (w588:dbl[])
      n286 = Array Subset(array=w589, index=10, length=500) -> (w587:dbl[])
      n287 = Array Subset(array=w578, index=1942, length=11) -> (w581:dbl[])
      n288 = call-poly <vilib>:"RMS.vi"("X"=w588) -> ("rms value"=w570:dbl)  [unwired: 1 out]
      n289 = Array Subset(array=w578, index=6037, length=11) -> (w579:dbl[])
      n290 = call <vilib>:"Std Deviation and Variance.vi"("X"=w587) -> ("standard deviation"=w586:dbl)  [unwired: 1 in, 2 out]
      n291 = call-poly <vilib>:"RMS.vi"("X"=w581) -> ("rms value"=w576:dbl)  [unwired: 1 out]
      n292 = call-poly <vilib>:"RMS.vi"("X"=w579) -> ("rms value"=w575:dbl)  [unwired: 1 out]
      n293 = Multiply(x=w586, y=w585) -> (x*y=w571:dbl)
      n294 = Divide(x=w571, y=w570) -> (x/y=w584:dbl)
      n295 = Add(x=w576, y=w575) -> (x+y=w577:dbl)
      n296 = Divide(x=w577, y=2.0) -> (x/y=w572:dbl)
      n297 = Divide(x=w572, y=w571) -> (x/y=w574:dbl)
      n298 = Build Array(w568, w592) -> (→"Current (Re and Im), Gaussian FFT vs Fit":dbl[][])
    }
    frame #5 {
      # "V1 Re/Im"
      # "V2 Re/Im"
      # "V3 Re/Im"
      # "V4 Re/Im"
      # "V5 Re/Im"
      # "Mag\n16-20"
      # "Phase\n16-20"
      # "Voltage 5th Im"
      # "Voltage 5th Real"
      # "Voltage 4th Im"
      # "Voltage 4th Re"
      # "Voltage 3rd Im"
      # "Voltage 3rd Real"
      # "Voltage 2nd Im"
      # "Voltage 2nd Real"
      # "Voltage 1st Im"
      # "Voltage 1st Real"
      # "Current 1st Imag"
      # "Current 1st Real"
      n299 = Index Array(array=w618, index=0) -> (element=w614:dbl)
      n300 = Index Array(array=w618, index=1) -> (element=w613:dbl)
      n301 = Index Array(array=w618, index=2) -> (element=w612:dbl)
      n302 = Index Array(array=w618, index=3) -> (element=w611:dbl)
      n303 = Index Array(array=w618, index=4) -> (element=w610:dbl)
      n304 = Index Array(array=w618, index=6) -> (element=w608:dbl)
      n305 = Index Array(array=w618, index=5) -> (element=w609:dbl)
      n306 = Index Array(array=w618, index=7) -> (element=w607:dbl)
      n307 = Index Array(array=w618, index=8) -> (element=w606:dbl)
      n308 = Index Array(array=w618, index=9) -> (element=w605:dbl)
      n309 = Index Array(array=w617, index=1) -> (element=w615:dbl)
      n310 = Index Array(array=w617, index=0) -> (element=w616:dbl)
      n311 = stacked-sequence {
        seq-local: [w653 _ _ _ _ _] -> [_ w670 w680 w690 w702 w714]
        tunnel: "Char Current (Amps)" -> [w659 _ _ _ _ _]
        tunnel: [w658 _ _ _ _ _] -> w652
        tunnel: [_ w668 _ _ _ _] -> w651
        tunnel: [_ w667 _ _ _ _] -> w650
        tunnel: [_ _ w678 _ _ _] -> w649
        tunnel: [_ _ w677 _ _ _] -> w648
        tunnel: [_ _ _ w688 _ _] -> w646
        tunnel: [_ _ _ w687 _ _] -> w645
        tunnel: [_ _ _ _ w700 _] -> w644
        tunnel: [_ _ _ _ w699 _] -> w643
        tunnel: [_ _ _ _ _ w712] -> w642
        tunnel: [_ _ _ _ _ w711] -> w641
        tunnel: [_ w666 _ _ _ _] -> w640
        tunnel: [_ _ w676 _ _ _] -> w639
        tunnel: [_ _ _ w686 _ _] -> w638
        tunnel: [_ _ _ _ w698 _] -> w637
        tunnel: [_ _ _ _ _ w710] -> w636
        tunnel: [_ w665 _ _ _ _] -> w635
        tunnel: [_ _ w672 _ _ _] -> w634
        tunnel: [_ _ _ w693 _ _] -> w633
        tunnel: [_ _ _ _ w705 _] -> w632
        tunnel: [_ _ _ _ _ w717] -> w631
        tunnel: w616 -> [w657 _ _ _ _ _]
        tunnel: w615 -> [w656 _ _ _ _ _]
        tunnel: w614 -> [_ w664 _ _ _ _]
        tunnel: w613 -> [_ w663 _ _ _ _]
        tunnel: w612 -> [_ _ w675 _ _ _]
        tunnel: w611 -> [_ _ w674 _ _ _]
        tunnel: w610 -> [_ _ _ w685 _ _]
        tunnel: w609 -> [_ _ _ w684 _ _]
        tunnel: w608 -> [_ _ _ _ w697 _]
        tunnel: w607 -> [_ _ _ _ w696 _]
        tunnel: w606 -> [_ _ _ _ _ w709]
        tunnel: w605 -> [_ _ _ _ _ w708]
        frame #0 {
          # "alpha"
          n312 = Re/Im To Complex(1:w656, 2:w657) -> (0:w661:cdb)
          n313 = Complex To Polar(r * e^(i*theta)=w661) -> (r=w660:dbl, theta=w653:dbl)
          "Current Amplitude" <- w660
          n314 = Divide(x=w660, y=w659) -> (x/y=w658:dbl)
          n315 = Multiply(x=w653, y=57.3) -> (x*y=→"Current Phase Correction":dbl)
        }
        frame #1 {
          n316 = Re/Im To Complex(1:w663, 2:w664) -> (0:w671:cdb)
          n317 = Complex To Polar(r * e^(i*theta)=w671) -> (r=w666:dbl, theta=w662:dbl)
          "V1 Amplitude" <- w666
          n318 = Subtract(x=w662, y=w670) -> (x-y=w665:dbl)
          n319 = Polar To Complex(1:w665, 2:w666) -> (0:w669:cdb)
          n320 = Complex To Re/Im(x + iy=w669) -> (x=w668:dbl, y=w667:dbl)
        }
        frame #2 {
          n321 = Re/Im To Complex(1:w674, 2:w675) -> (0:w683:cdb)
          n322 = Complex To Polar(r * e^(i*theta)=w683) -> (r=w676:dbl, theta=w673:dbl)
          n323 = Multiply(x=w680, y=2.0) -> (x*y=w679:dbl)
          n324 = Subtract(x=w673, y=w679) -> (x-y=w672:dbl)
          n325 = Polar To Complex(1:w672, 2:w676) -> (0:w682:cdb)
          n326 = Complex To Re/Im(x + iy=w682) -> (x=w678:dbl, y=w677:dbl)
        }
        frame #3 {
          n327 = Re/Im To Complex(1:w684, 2:w685) -> (0:w695:cdb)
          n328 = Complex To Polar(r * e^(i*theta)=w695) -> (r=w686:dbl, theta=w694:dbl)
          n329 = Multiply(x=w690, y=3.0) -> (x*y=w689:dbl)
          n330 = Subtract(x=w694, y=w689) -> (x-y=w693:dbl)
          n331 = Polar To Complex(1:w693, 2:w686) -> (0:w692:cdb)
          n332 = Complex To Re/Im(x + iy=w692) -> (x=w688:dbl, y=w687:dbl)
        }
        frame #4 {
          n333 = Re/Im To Complex(1:w696, 2:w697) -> (0:w707:cdb)
          n334 = Complex To Polar(r * e^(i*theta)=w707) -> (r=w698:dbl, theta=w706:dbl)
          n335 = Multiply(x=w702, y=4.0) -> (x*y=w701:dbl)
          n336 = Subtract(x=w706, y=w701) -> (x-y=w705:dbl)
          n337 = Polar To Complex(1:w705, 2:w698) -> (0:w704:cdb)
          n338 = Complex To Re/Im(x + iy=w704) -> (x=w700:dbl, y=w699:dbl)
        }
        frame #5 {
          n339 = Re/Im To Complex(1:w708, 2:w709) -> (0:w719:cdb)
          n340 = Complex To Polar(r * e^(i*theta)=w719) -> (r=w710:dbl, theta=w718:dbl)
          n341 = Multiply(x=w714, y=5.0) -> (x*y=w713:dbl)
          n342 = Subtract(x=w718, y=w713) -> (x-y=w717:dbl)
          n343 = Polar To Complex(1:w717, 2:w710) -> (0:w716:cdb)
          n344 = Complex To Re/Im(x + iy=w716) -> (x=w712:dbl, y=w711:dbl)
        }
      }
    }
  }
  n345 = property on="Current (Re and Im), Gaussian FFT vs Fit" class="WFGraph (strict)"("BG Color"=w5) -> ()  [unwired: 2 in, 2 out]
  n346 = property on="Voltage (Re and Im), Gaussian FFT vs Fit" class="WFGraph (strict)"("BG Color"=w5) -> ()  [unwired: 2 in, 2 out]
  n347 = Build Array(w40, w41, w42, w43, w44, w45, w46, w47, w48, w49, w50, w51, w52, w53, w54, w55, w56, w57, w58, w59, w60, w13, w12, w19, w18, w17, w16, w15, w14, w11, w10, w9, w8) -> (→"Fit Coefficients and Noise Ratios":dbl[])
